vi "SwerveDriveClose.vi"(8 "error in (no error)":errorcluster, 11 "SwerveDriveDevRef":T1={"DevStatus"={"status"=FALSE, "code"=0, "source"=""}, "TurnMotors[]"=[], "Square Inputs"=FALSE, "Max Output"=1.0, "DriveMotors[]"=[], "WheelOffset[]"=[], "SwerveSensors[]"=[], "RobotSize"={"Width"=[], "Length"=[], "Center"=[]}}) -> (0 "error out":errorcluster)   [LabVIEW 2019, in "Swerve Drive.lvlib"]
doc: "Closes the reference to the robot drive you specify. Use this VI to close each robot drive reference that you open with the Open2Motor VI or the Open4Motor VI.\n\nThis software is licensed. Open the labview\\readme\\WPI Robotics Library Open Source License.txt file for more information."
uses:
  Swerve Drive.lvlib
  SwerveDriveDevRef.ctl
  <vilib>/Rock Robotics/WPI/MotorControl/WPI_MotorControlDeviceRef.ctl
  <vilib>/Rock Robotics/WPI/MotorControl/WPI_MotorControlType.ctl
  <vilib>/Rock Robotics/SystemInterfaces/DIO/FPGA_DIOPWMChannel.ctl
  <vilib>/Rock Robotics/WPI/PWM/WPI_PWMDeadband.ctl
  <vilib>/Rock Robotics/SystemInterfaces/DIO/FPGA_DIOChannel.ctl
  <vilib>/Rock Robotics/SystemInterfaces/AI/FPGA_AIChannel.ctl
  <vilib>/Rock Robotics/WPI/SafetyOutput/WPI_SafetyOutputConfigMenu.ctl
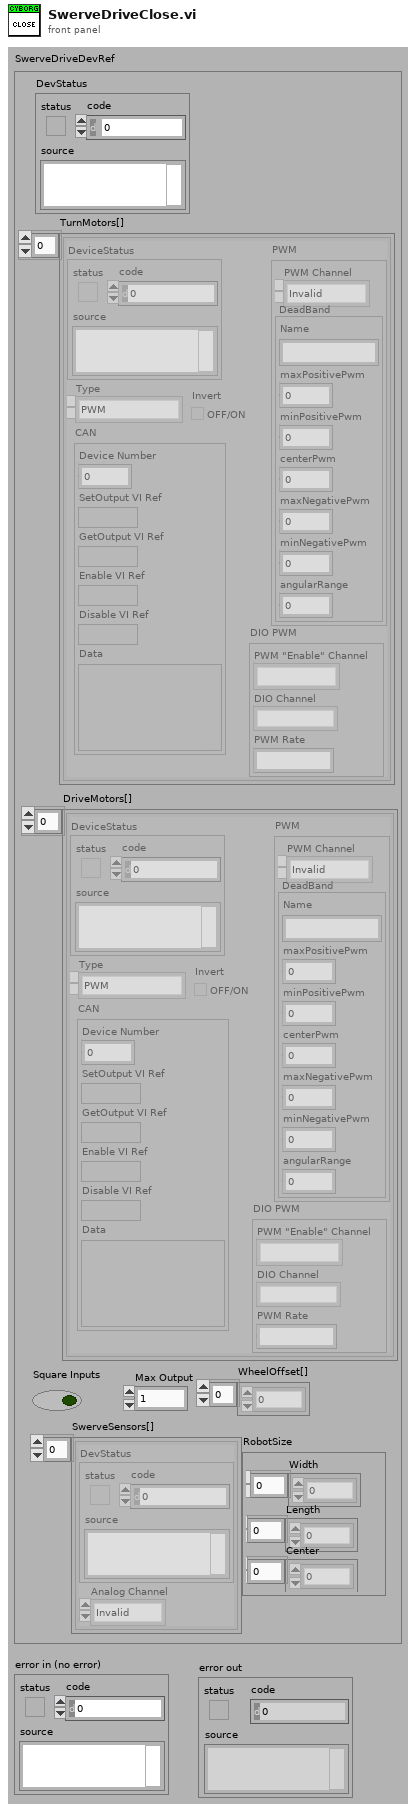
[diagram p1: front panel]
types:
  T1 = typedef "Swerve Drive.lvlib/SwerveDriveDevRef.ctl" = cluster{"DevStatus":errorcluster, "TurnMotors[]":T2[], "Square Inputs":bool, "Max Output":dbl, "DriveMotors[]":T2[], "WheelOffset[]":dbl[], "SwerveSensors[]":cluster{"DevStatus":errorcluster, "Analog Channel":T7}[], "RobotSize":cluster{"Width":dbl[], "Length":dbl[], "Center":dbl[]}}
  T2 = typedef "WPI_MotorControlDeviceRef.ctl" = cluster{"DeviceStatus":errorcluster, "Type":T3, "PWM":cluster{"PWM Channel":T4, "DeadBand":T5}, "CAN":cluster{"Device Number":u8, "SetOutput VI Ref":variant, "GetOutput VI Ref":variant, "Enable VI Ref":variant, "Disable VI Ref":variant, "Data":variant}, "Invert":bool, "DIO PWM":cluster{"PWM \"Enable\" Channel":T4, "DIOChannel":T6, "PWM Rate":dbl}}
  T3 = typedef "WPI_MotorControlType.ctl" = enum16{"PWM", "CAN", "DIO PWM"}
  T4 = typedef "FPGA_DIOPWMChannel.ctl" = enum8{"PWM 0", "PWM 1", "PWM 2", "PWM 3", "PWM 4", "PWM 5", "PWM 6", "PWM 7", "PWM 8", "PWM 9", "PWM MXP 0", "PWM MXP 1", "PWM MXP 2", "PWM MXP 3", "PWM MXP 4", "PWM MXP 5", "PWM MXP 6", "PWM MXP 7", "PWM MXP 8", "PWM MXP 9", "Invalid"}
  T5 = typedef "WPI_PWMDeadband.ctl" = cluster{"Name":string, "maxPositivePwm":i32, "minPositivePwm":i32, "centerPwm":i32, "maxNegativePwm":i32, "minNegativePwm":i32, "angularRange":u16}
  T6 = typedef "FPGA_DIOChannel.ctl" = enum8{"DIO 0", "DIO 1", "DIO 2", "DIO 3", "DIO 4", "DIO 5", "DIO 6", "DIO 7", "DIO 8", "DIO 9", "DIO MXP 0", "DIO MXP 1", "DIO MXP 2", "DIO MXP 3", "DIO MXP 4", "DIO MXP 5", "DIO MXP 6", "DIO MXP 7", "DIO MXP 8", "DIO MXP 9", "DIO MXP 10", "DIO MXP 11", "DIO MXP 12", "DIO MXP 13", "DIO MXP 14", "DIO MXP 15", "SPI Port CS1", "SPI Port CS2", "SPI Port CS3", "SPI Port MISO", "SPI Port MOSI", "Invalid"}
  T7 = typedef "FPGA_AIChannel.ctl" = enum8{"AI 0", "AI 1", "AI 2", "AI 3", "AI MXP 0", "AI MXP 1", "AI MXP 2", "AI MXP 3", "Invalid"}
  T8 = typedef "WPI_SafetyOutputConfigMenu.ctl" = enum16{"Enable", "Disable"}
  T9 = cluster{"DevStatus":errorcluster, "Analog Channel":T7}[]
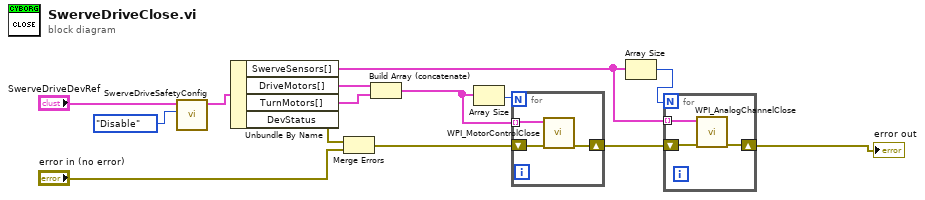
[diagram p0: block diagram]
diagram:
  n1 = call "SwerveDriveSafetyConfig.vi"("mode"=WPI_SafetyOutputConfigMenu."Disable", "SwerveDriveDevRef"="SwerveDriveDevRef") -> ("SwerveDriveDevRef"=w8:T1)  [unwired: 8 in, 1 out]
  n2 = Unbundle By Name(w8) -> ("SwerveSensors[]"=w1:T9, "DriveMotors[]"=w5:T2[], "TurnMotors[]"=w14:T2[], "DevStatus"=w12:errorcluster)
  n3 = Merge Errors(w12, "error in (no error)") -> (w10:errorcluster)
  n4 = Build Array (concatenate)(w5, w14) -> (w6:T2[])
  n5 = Array Size(array=w6) -> (size(s)=w13:i32)
  n6 = for {
    N: w13 -> [_]
    tunnel: w6 -> [w15] mode=indexing
    shift-right: [w17] -> w3
    shift-left: w10 -> [w16]
    n7 = call <vilib>:"WPI_MotorControlClose.vi"("error in"=w16, "MotorControlDevRef"=w15) -> ("error out"=w17:errorcluster)  [unwired: 9 out]
  }
  n8 = Array Size(array=w1) -> (size(s)=w2:i32)
  n9 = for {
    N: w2 -> [_]
    shift-right: [w20] -> w4
    shift-left: w3 -> [w19]
    tunnel: w1 -> [w18] mode=indexing
    n10 = call <vilib>:"WPI_AnalogChannelClose.vi"("error in (no error)"=w19, "AIDeviceRef"=w18) -> ("error out"=w20:errorcluster)  [unwired: 9 in]
  }
  "error out" <- w4
